vi "Synthetic_Jet_Measurement_v2.vi"() -> (5 "Plug in titles":string[](array[string]), 7 "Plug in values":string[](array[string]))   [LabVIEW 2011]
uses:
  Controls/SJ_Channels.ctl
  Controls/SJ_Data_Cluster.ctl
  <vilib>/Analysis/2dsp.llb/Integral Method.ctl
  Globals/Meas_global.vi
  Globals/Plug_in_data_global.vi
  <vilib>/Analysis/baseanly.llb/Scale 1D.vi
  <vilib>/Analysis/5stat.llb/RMS (DBL).vi
  <vilib>/Analysis/8numeric.llb/1D Numeric Integration.vi
  <vilib>/Analysis/baseanly.llb/Quick Scale 1D.vi
  <vilib>/Analysis/1siggen.llb/Ramp Pattern by Samples.vi
  <vilib>/Analysis/NI_AALBase.lvlib
  <vilib>/Analysis/NI_AALPro.lvlib
panel:
  out "Phase Average?":bool
  out "Samps per cyle":i32
  in  "Synthetic Jet Specific Channels":T1=["Synthetic_Jet:Orifice:Volume", "Synthetic_Jet:Orifice:Height", "Synthetic_Jet:Orifice:Diameter", "Synthetic_Jet:Cavity:Volume", "Synthetic_Jet:Cavity:Height", "Synthetic_Jet:Cavity:Diameter", "Synthetic_Jet:Samples:Per_Cycle", "Synthetic_Jet:Dwell:Time", "Synthetic_Jet:Minimum:Frequency", "Synthetic_Jet:Maximum:Frequency", "Synthetic_Jet:Minimum:Amplitude", "Synthetic_Jet:Maximum:Amplitude", "Synthetic_Jet:Amplitude:Delta", "Synthetic_Jet:Frequency:Delta", "Synthetic_Jet:Calibration:Velocity", "Synthetic_Jet:Calibration:Max_Amplitude", "Synthetic_Jet:Calibration:Active?", "Synthetic_Jet:Calibration:No_Of_Gens", "Synthetic_Jet:Optimisation:Switch", "Synthetic_Jet:Identification:Number"]
  out "Formation Criteria":dbl
  out "Jet Formation":bool
  out "Strouhal Number":dbl
  out "Stokes Number":dbl
  out "nu":dbl=1.55e-05
  out "Omega":dbl=1200.0
  out "Reynolds Number":dbl
  out "Charicteristic Velocity m_s":dbl
  out "Stroke Length _m_":dbl
  out "DL:Frequency":dbl=2.802671520827615
  out "Cavity:Helmholtz:Hz":dbl=428.16291209383184
  out "DL:Radius":dbl
  out "DL:Streamwise:Position":dbl=5.0
  out "LEM Velocity _ms_":dbl[](array[numeric])=[3.7049856348371377, 3.4607988115264297, 3.0653584733968287, 2.5359472607578692, 1.895702983998723, 1.1726073902466658, 0.3982632267462864, -0.3934869508418966, -1.1680398605184126, -1.8915438234131698, -2.5323782445904723, -3.062535584780142, -3.458845424238726, -3.7039871212762807, -3.787246807411894, -3.7049856348371377, -3.4607988115264297, -3.0653584733968295, -2.5359472607578692, -1.8957029839987247, -1.172607390246666, -0.3982632267462887, 0.3934869508418962, 1.1680398605184101, 1.8915438234131694, 2.53237824459047, 3.0625355847801417, 3.4588454242387248, 3.7039871212762803, 3.7872468074118935]
  out "LEM Max Velocity _ms_":dbl=3.7872475686779676
  out "LEM Phase Velocity _deg_":dbl=-258.0363282123533
  out "Phase Power _deg_":dbl=-1216.295394809798
  out "Phase Current _deg_":dbl=114.2968039724566
  out "RV Phase Pressure _deg_":dbl
  out "Phase Pressure _deg_":dbl=-169.14507601114087
  out "Phase Displ _deg_":dbl=-40.709415815185025
  out "Phase Velocity _deg_":dbl=373.1272896341652
  out "Phase Input Voltage _deg_":dbl=8.606071626556414
  out "Phase Angle _deg_":dbl[](array[numeric])=[0.0, 12.0, 24.0, 36.0, 48.0, 60.0, 72.0, 84.0, 96.0, 108.0, 120.0, 132.0, 144.0, 156.0, 168.0, 180.0, 192.0, 204.0, 216.0, 228.0, 240.0, 252.0, 264.0, 276.0, 288.0, 300.0, 312.0, 324.0, 336.0, 348.0]
  out "Max Power _W_":dbl=0.09567394666235574 format="%0.2f"
  out "Amplitude (V)":dbl=70.0
  out "Frequency (Hz)":dbl=1200.0
  out "AS Freq":dbl=36036.04
  out "Output Data Names":string[](array[string])=["Max Pressure _Pa_", "Max Velocity m_s", "Max Current _A_", "Max Displacement _m_", "Phase Displ _deg_", "Phase Pressure _deg_", "Phase Velocity _deg_", "Phase Current _deg_", "Phase Input Voltage _deg_", "LEM Max Velocity _ms_", "LEM Phase Velocity _deg_"]
  out "Current _A_":dbl[](array[numeric])=[0.007871578951352444, 0.008266417140890889, 0.00849968074403876, 0.008455354076272185, 0.007734598407207069, 0.006567672714377243, 0.00502412226480415, 0.003160545427498193, 0.0011561900642313688, -0.0008322812950871137, -0.0026496409136783387, -0.004250177970402979, -0.0056599044207173484, -0.006974613805967722, -0.007544462997563997, -0.008243629249997945, -0.008448348909812501, -0.008596065082556333, -0.008270248882544743, -0.007591372292965107, -0.0065346555924612445, -0.005182607825984795, -0.003607407527949277, -0.0016626720392260718, 0.00036386353784322137, 0.0021437834956932957, 0.003704399543557329, 0.005128068807114345, 0.006438338773620389, 0.007353635511234548]
  out "Power_W_":dbl[](array[numeric])=[-0.043363451952469156, -0.1045787042911587, -0.16349661489678932, -0.21135096948039916, -0.2294893577920496, -0.21702510361561647, -0.17587031608696657, -0.11191242161210375, -0.03966959410717387, 0.026383849953920794, 0.07342545396353153, 0.09567394666235574, 0.0925358489049179, 0.06622858320017053, 0.01657193795313242, -0.042740863570043953, -0.10421979243576313, -0.16261661392816973, -0.2041915474460092, -0.22315321729709184, -0.2143088761872366, -0.18014115682356102, -0.12703551569073906, -0.05674338994484436, 0.011476164341731257, 0.059131235834024416, 0.08299512964242624, 0.08340916969883025, 0.06053396412209597, 0.01568890358261011]
  out "RV Pressure _V_":dbl[](array[numeric])=[-14.369666524328046, -57.77058962565634, -87.07652966541758, -117.51006835010423, -142.3114261743131, -158.09199483911908, -155.83679754926837, -151.8902022920296, -142.3114261743131, -120.32906496241762, -88.20412831034297, -49.31359978871612, -12.114469234477319, 29.02544421285115, 67.35217341201532, 101.7323073539407, 128.78305010385122, 147.3826153809706, 157.5310031852989, 162.59938472331393, 149.63781267082135, 136.11244129586606, 102.29610667640338, 72.99016663664214, 42.55081558780641, -5.354689729074237, -48.18600114379076, -84.25753305310417, -116.38246970517886, -138.36483091707433, -158.65579416158175, -165.41557366698484, -160.34719212896982, -149.0712056797162, -122.58426225226835, -92.71452289004439, -56.642990980730964, -17.188663136641456, 24.515049633149694, 61.15038086492581, 97.22191277423924, 132.1658460386273, 151.3292106382094, 160.34418743346322, 160.34418743346322, 155.27580589544817, 136.67624061832876, 106.80650125610484, 74.67575223988108, 33.5358387925526, -1.9718937942981463, -42.553820283313044, -85.38513169802953, -116.38246970517886, -141.74762685185044, -159.78339280650712, -164.28797502205947, -162.03859009635784, -141.18382752938774, -123.71186089719372, -94.40592085743245, -59.46198759304437, -20.007659748954865, 21.70186538498539, 58.3313842526124, 92.14771887207513, 124.27846788829885, 149.63781267082135, 160.34418743346322, 156.9672038628362, 155.27580589544817, 141.75043452049292, 110.18348482673184, 77.49474885219449, 41.987016265343726, 0.2833034955525799, -41.42622163838768, -76.37015490277572, -109.62269019977577, -131.59923904752216, -159.21959348404445, -167.67077095683558, -160.9109914514325, -151.8902022920296, -125.96705818704444, -102.29329900776088, -63.96656980859674, -33.53303112391013, 16.627671482821253, 53.82680203706004, 93.27531751700047, 122.58706992091082, 148.51021402589598, 158.65860183022428, 155.27580589544817, 156.9672038628362, 142.30842147880648, 120.3318726310601, 80.31374546450789, 48.18880881243323, 10.425878935731753, -34.6606297688355, -76.37015490277572, -108.49509155485042, -133.85443633737287, -151.8902022920296, -162.03859009635784, -164.28797502205947, -154.709198904343, -135.54583430476092, -104.54849629761163, -71.85976032307427, -32.96923180144745, 7.0430830009556615, 52.135404069672006, 85.95173868913471, 118.64047466367205, 142.30842147880648, 157.5310031852989, 159.78038811100052, 158.09480250776156, 142.30842147880648, 123.71466856583618, 86.5155380115974, 49.316407457358586, 13.244875548045162, -27.33705094096973, -69.04076371076087, -103.42089765268625, -130.4716404025968, -151.8902022920296, -160.34719212896982, -162.60238941882054, -154.14539958188033, -135.54583430476092, -104.54849629761163, -71.85976032307427, -36.91582705868622, 4.793698075254034, 51.007805424746635, 81.44134410943326, 115.82147805135864, 140.62283587556755, 154.1482072505228, 160.9079867559259, 156.40340454037351, 145.69121741358256, 120.89567195352278, 93.27531751700047, 54.95440068198541]
  out "Displacement _m_":dbl[](array[numeric])=[-2.6563452608725367e-05, -3.3033094590941884e-05, -3.489470009695634e-05, -3.608459414033635e-05, -3.599336290251176e-05, -3.300271431749379e-05, -3.056117109155232e-05, -2.2626856342716373e-05, -1.762170629215838e-05, -1.0755312405507711e-05, -5.5370483534114006e-06, -2.8768068802271785e-07, 4.656075893275746e-06, 8.287603580077764e-06, 1.4940431377787088e-05, 1.9792866303780654e-05, 2.4126214474223672e-05, 2.519431617137013e-05, 2.644560368400959e-05, 2.7208727219429685e-05, 2.372973382223118e-05, 2.04641256790127e-05, 1.719906004067715e-05, 1.3689415117589209e-05, 8.043566800208257e-06, 4.4422385518931854e-06, -1.2338996214552368e-06, -5.841845680176716e-06, -1.1396101089811283e-05, -1.6401251140369278e-05]
  out "Input Voltage _V_":dbl[](array[numeric])=[-5.5088632433799996, -12.651031578584, -19.235618350895997, -24.9961110527, -29.670494279084004, -33.04444558276, -35.005182361704, -35.409211536216006, -34.310616683552006, -31.700640287920002, -27.711473499856005, -22.510574222680006, -16.349366000988, -9.495663135284, -2.196569584672, 5.184714435096, 12.336113665324001, 18.917564300223997, 24.689891482827996, 29.395636083331993, 32.795741589576, 34.758786092276, 35.215182844328, 34.127830748423996, 31.539748142271996, 27.582652797175996, 22.404475723135995, 16.265220463328, 9.402109185388, 2.133489422836]
  out "Pressure _Pa_":dbl[](array[numeric])=[-27.3956675953706, 95.65286233449294, 217.28142105099454, 325.3916285730047, 412.49320713856633, 477.62511872885386, 518.8812420389512, 544.5955786383588, 546.2858417945154, 525.7943338813993, 485.98446016799124, 431.53940396868336, 357.29264741860004, 257.81676584697294, 146.44897730607346, 25.39291194062997, -95.29994862668336, -216.63005998968256, -325.4638615668826, -412.65459893301875, -477.423305725176, -519.6780076017092, -543.7330519967387, -544.6659346048561, -524.568602441649, -487.2326508157636, -435.0203186855821, -361.9795522274816, -267.2741357434412, -152.01151538796677]
  out "Zeros":dbl[](array[numeric])=[1.4978743085562871, 0.2341330189017041, -0.35175473981443495, 0.0022887999999999997, -3.0068544366899315, 2.8293]
  out "Velocity m_s":dbl[](array[numeric])=[-0.006589971422005106, -0.006419643065741468, -0.009111611844261746, -0.006030326884042168, -0.004272653157727323, -0.0068849933436421745, -0.010636233235274354, -0.0035467148583991693, -0.008496862890472292, -0.005357351691532665, -0.007065956289182962, -0.006648911559621155, -0.005058171342073957, -0.008830133605031026, -0.0038751674420970687, -0.005274584307176274, 0.000979796600094568, -0.005616008146962059, -0.00729733372181674, 0.0005036149760482819, -0.004633370846616606, -0.007598533001820504, -0.005354959759266961, -0.003855515705978843, -0.005082756078867318, -0.0008163141834672163, -0.007346968606858383, -0.00413574997102441, -0.00277648312445221, -0.00052352239052674]
  out "Max Current _A_":dbl=0.00849968074403876 format="%e"
  out "RMS Dispacement _m_":dbl=2.25005755896471e-05 format="%0.2f"
  out "RMS Velocity m_s":dbl=0.014914535983039488 format="%0.2f"
  out "RMS Current _A_":dbl=0.006206722435388947 format="%0.2f"
  out "RV RMS Pressure _V_":dbl format="%0.2f"
  out "RMS Pressure _Pa_":dbl=395.7699897259115 format="%0.2f"
  out "RMS Power _W_":dbl=0.13002833315099252 format="%0.2f"
  out "Max Displacement _m_":dbl=2.7208727219429685e-05 format="%e"
  out "Max Pressure _Pa_":dbl=546.2858417945154 format="%0.2f"
  out "RV Max Pressure _V_":dbl format="%0.2f"
  out "Max Velocity m_s":dbl=0.000979796600094568
  out "Current Plot":cluster{dbl[], dbl[]}[](graph)=[{[0.0, 12.0, 24.0, 36.0, 48.0, 60.0, 72.0, 84.0, 96.0, 108.0, 120.0, 132.0, 144.0, 156.0, 168.0, 180.0, 192.0, 204.0, 216.0, 228.0, 240.0, 252.0, 264.0, 276.0, 288.0, 300.0, 312.0, 324.0, 336.0, 348.0], [-0.15557712257291065, -0.35728080433659803, -0.5432376920119246, -0.705921142218441, -0.8379315153272326, -0.9332160799164545, -0.9885897155857659, -1.0, -0.9689743203815658, -0.8952653536353687, -0.7826063416157439, -0.6357265029653804, -0.4617263500562873, -0.2681692905127802, -0.06203384626131485, 0.1464227586596542, 0.34838713233438734, 0.5342554516040381, 0.697273122209331, 0.8301691793748806, 0.926192371045399, 0.9816311796924717, 0.9945203893712923, 0.9638122191316959, 0.8907215601232357, 0.7789682853842954, 0.632730149899583, 0.45934997583022086, 0.26552721106968635, 0.060252384345070756]}, {[0.0, 12.0, 24.0, 36.0, 48.0, 60.0, 72.0, 84.0, 96.0, 108.0, 120.0, 132.0, 144.0, 156.0, 168.0, 180.0, 192.0, 204.0, 216.0, 228.0, 240.0, 252.0, 264.0, 276.0, 288.0, 300.0, 312.0, 324.0, 336.0, 348.0], [0.915718863893427, 0.9616512975995976, 0.9887873884629885, 0.9836307653638304, 0.8997836024883751, 0.7640324556993839, 0.5844676856855597, 0.36767351074525567, 0.13450224644966696, -0.09682119517406056, -0.3082388148799797, -0.49443296782707047, -0.6584296845544803, -0.8113728478069623, -0.8776647134598465, -0.9590003298982027, -0.9828158382556238, -1.0, -0.962097052909388, -0.8831217795651628, -0.7601914980520298, -0.6029046751288172, -0.41965800552972216, -0.19342245821289428, 0.04232908131205239, 0.24939125926856856, 0.4309413095387709, 0.5965600257634787, 0.7489867412341333, 0.855465313560387]}]
  in  "Menu Ring":u16(ring) items=["Max Pressure _Pa_", "Max Velocity m_s", "Max Current _A_", "Max Displacement _m_", "Phase Displ _deg_", "Phase Pressure _deg_", "Phase Velocity _deg_", "Phase Current _deg_", "Phase Input Voltage _deg_", "LEM Max Velocity _ms_", "LEM Phase Velocity _deg_"]
  out "Pressure v Frequency":cluster{dbl[], dbl[]}(graph)
  out "Pressure Plot":cluster{dbl[], dbl[]}[](graph)=[{[0.0, 12.0, 24.0, 36.0, 48.0, 60.0, 72.0, 84.0, 96.0, 108.0, 120.0, 132.0, 144.0, 156.0, 168.0, 180.0, 192.0, 204.0, 216.0, 228.0, 240.0, 252.0, 264.0, 276.0, 288.0, 300.0, 312.0, 324.0, 336.0, 348.0], [-0.15557712257291065, -0.35728080433659803, -0.5432376920119246, -0.705921142218441, -0.8379315153272326, -0.9332160799164545, -0.9885897155857659, -1.0, -0.9689743203815658, -0.8952653536353687, -0.7826063416157439, -0.6357265029653804, -0.4617263500562873, -0.2681692905127802, -0.06203384626131485, 0.1464227586596542, 0.34838713233438734, 0.5342554516040381, 0.697273122209331, 0.8301691793748806, 0.926192371045399, 0.9816311796924717, 0.9945203893712923, 0.9638122191316959, 0.8907215601232357, 0.7789682853842954, 0.632730149899583, 0.45934997583022086, 0.26552721106968635, 0.060252384345070756]}, {[0.0, 12.0, 24.0, 36.0, 48.0, 60.0, 72.0, 84.0, 96.0, 108.0, 120.0, 132.0, 144.0, 156.0, 168.0, 180.0, 192.0, 204.0, 216.0, 228.0, 240.0, 252.0, 264.0, 276.0, 288.0, 300.0, 312.0, 324.0, 336.0, 348.0], [-0.05014896140338823, 0.1750967259562854, 0.39774309423293575, 0.5956435325215701, 0.7550867615085017, 0.8743135592895557, 0.9498346878887768, 0.9969058997564276, 1.0, 0.9624894032658751, 0.8896156974736197, 0.7899516534258018, 0.6540397353973438, 0.47194480640402603, 0.2680812243366908, 0.0464828300459258, -0.17445070206035157, -0.39655074947222896, -0.5957757581594167, -0.7553821962097238, -0.87394413180629, -0.9512932019153176, -0.9953270072140422, -0.9970346894139926, -0.9602456485390019, -0.8919005647578826, -0.7963236192550169, -0.6626193185574809, -0.4892569334498257, -0.2782636922981901]}]
  out "Displacement Plot":cluster{dbl[], dbl[]}[](graph)=[{[0.0, 12.0, 24.0, 36.0, 48.0, 60.0, 72.0, 84.0, 96.0, 108.0, 120.0, 132.0, 144.0, 156.0, 168.0, 180.0, 192.0, 204.0, 216.0, 228.0, 240.0, 252.0, 264.0, 276.0, 288.0, 300.0, 312.0, 324.0, 336.0, 348.0], [-0.15557712257291065, -0.35728080433659803, -0.5432376920119246, -0.705921142218441, -0.8379315153272326, -0.9332160799164545, -0.9885897155857659, -1.0, -0.9689743203815658, -0.8952653536353687, -0.7826063416157439, -0.6357265029653804, -0.4617263500562873, -0.2681692905127802, -0.06203384626131485, 0.1464227586596542, 0.34838713233438734, 0.5342554516040381, 0.697273122209331, 0.8301691793748806, 0.926192371045399, 0.9816311796924717, 0.9945203893712923, 0.9638122191316959, 0.8907215601232357, 0.7789682853842954, 0.632730149899583, 0.45934997583022086, 0.26552721106968635, 0.060252384345070756]}, {[0.0, 12.0, 24.0, 36.0, 48.0, 60.0, 72.0, 84.0, 96.0, 108.0, 120.0, 132.0, 144.0, 156.0, 168.0, 180.0, 192.0, 204.0, 216.0, 228.0, 240.0, 252.0, 264.0, 276.0, 288.0, 300.0, 312.0, 324.0, 336.0, 348.0], [-0.7361438653132033, -0.9154348379941063, -0.9670248738630008, -1.0, -0.997471739948916, -0.9145929198799676, -0.8469312685822951, -0.6270503211070746, -0.48834431180314575, -0.2980582894650082, -0.15344632481876624, -0.00797239638899362, 0.12903223672595104, 0.2296715198692966, 0.4140390583217413, 0.5485129256769343, 0.668601519540294, 0.6982014560947281, 0.7328779584207091, 0.7540261396210363, 0.6576139870090829, 0.5671153068654675, 0.47663166097388826, 0.3793700731217815, 0.22290861216080401, 0.12310623571424707, -0.03419463765219268, -0.16189306875552578, -0.3158162468307329, -0.45452225613466185]}]
  out "Velocity Plot":cluster{dbl[], dbl[]}[](graph)=[{[0.0, 12.0, 24.0, 36.0, 48.0, 60.0, 72.0, 84.0, 96.0, 108.0, 120.0, 132.0, 144.0, 156.0, 168.0, 180.0, 192.0, 204.0, 216.0, 228.0, 240.0, 252.0, 264.0, 276.0, 288.0, 300.0, 312.0, 324.0, 336.0, 348.0], [-0.15557712257291065, -0.35728080433659803, -0.5432376920119246, -0.705921142218441, -0.8379315153272326, -0.9332160799164545, -0.9885897155857659, -1.0, -0.9689743203815658, -0.8952653536353687, -0.7826063416157439, -0.6357265029653804, -0.4617263500562873, -0.2681692905127802, -0.06203384626131485, 0.1464227586596542, 0.34838713233438734, 0.5342554516040381, 0.697273122209331, 0.8301691793748806, 0.926192371045399, 0.9816311796924717, 0.9945203893712923, 0.9638122191316959, 0.8907215601232357, 0.7789682853842954, 0.632730149899583, 0.45934997583022086, 0.26552721106968635, 0.060252384345070756]}, {[0.0, 12.0, 24.0, 36.0, 48.0, 60.0, 72.0, 84.0, 96.0, 108.0, 120.0, 132.0, 144.0, 156.0, 168.0, 180.0, 192.0, 204.0, 216.0, 228.0, 240.0, 252.0, 264.0, 276.0, 288.0, 300.0, 312.0, 324.0, 336.0, 348.0], [-0.0017400427690923374, -0.0016950685794170583, -0.002405866928563968, -0.0015922719565676093, -0.001128168660507009, -0.0018179415532591603, -0.002808434141249664, -0.0009364889690996669, -0.002243546122698781, -0.0014145768585897204, -0.0018657237429983216, -0.001755605561963586, -0.0013355800662831847, -0.0023315442732039188, -0.0010232149208002786, -0.001392722622896813, 0.00025870946624789303, -0.0014828735576385352, -0.0019268175782828233, 0.00013297653986074366, -0.0012234140213805954, -0.002006347457194939, -0.0014139452830977239, -0.0010180259967302217, -0.001342071519849202, -0.00021554290622666447, -0.0019399233745421283, -0.001092020188103525, -0.0007331138596561618, -0.00013823297428152076]}, {[0.0, 12.0, 24.0, 36.0, 48.0, 60.0, 72.0, 84.0, 96.0, 108.0, 120.0, 132.0, 144.0, 156.0, 168.0, 180.0, 192.0, 204.0, 216.0, 228.0, 240.0, 252.0, 264.0, 276.0, 288.0, 300.0, 312.0, 324.0, 336.0, 348.0], [0.9782794265180274, 0.9138033477917035, 0.8093896778519208, 0.6696017951074252, 0.5005491008108334, 0.3096200089077361, 0.10515903689372944, -0.10389788964157722, -0.3084139798421589, -0.49945089918916635, -0.6686594176102914, -0.8086443108979737, -0.9132875674934984, -0.9780157749495838, -1.0, -0.9782794265180274, -0.9138033477917035, -0.8093896778519211, -0.6696017951074252, -0.5005491008108338, -0.30962000890773617, -0.10515903689373006, 0.10389788964157712, 0.3084139798421583, 0.4994508991891662, 0.6686594176102908, 0.8086443108979736, 0.9132875674934979, 0.9780157749495837, 0.9999999999999999]}]
  out "Amplitude String":string="3.5000"
  out "Frequency String":string="1200"
  # "You Must have selected the \"Save Data\" option on the \nMeasurement Program for this vi to work correctly"
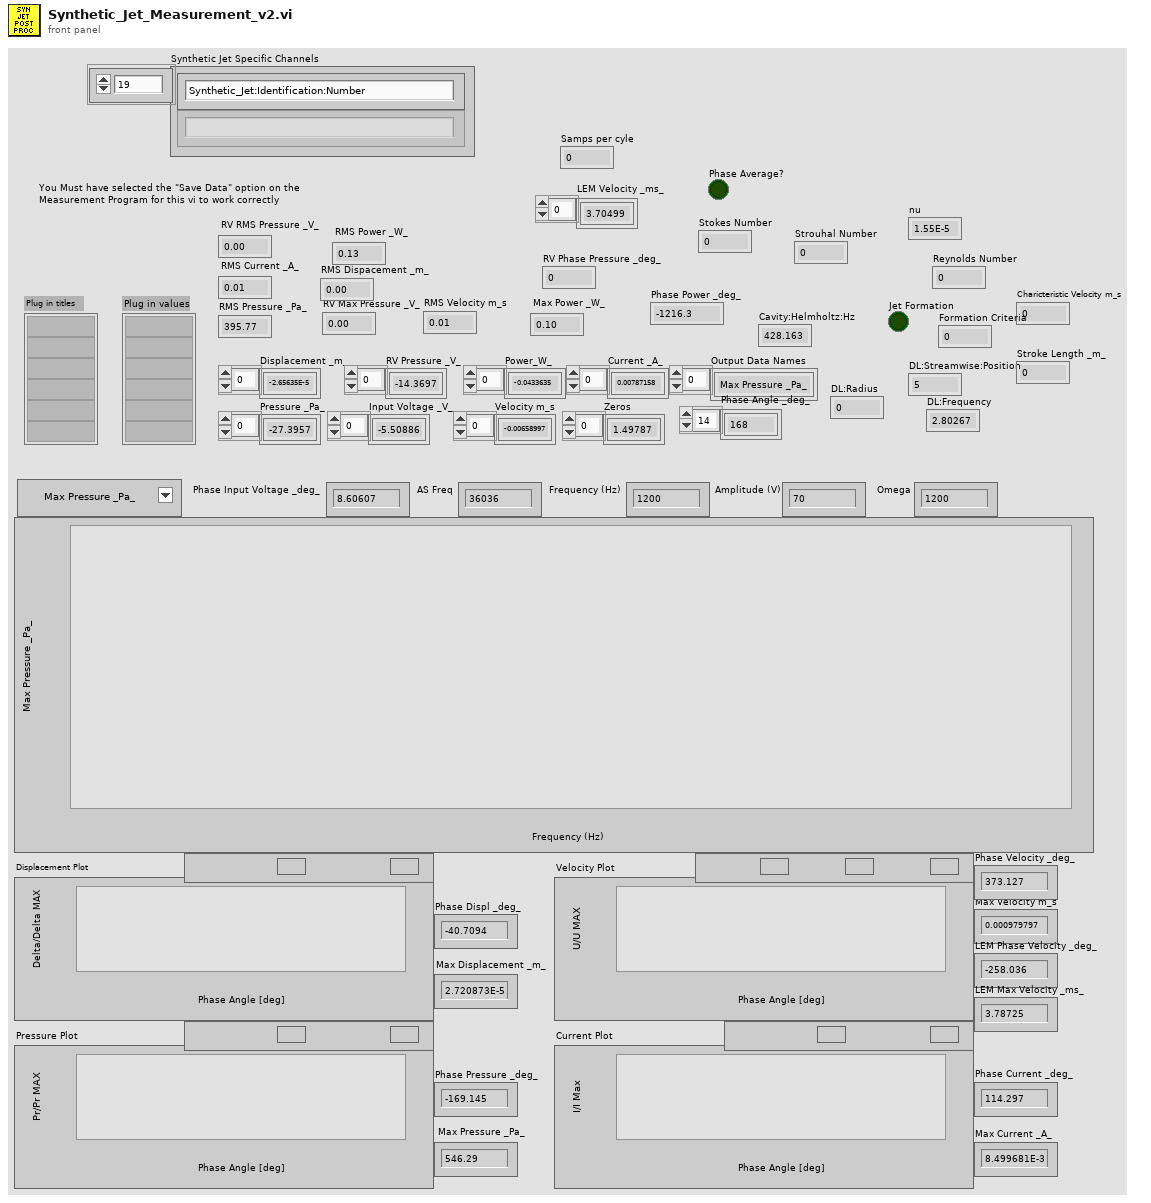
[diagram p1: front panel]
types:
  T1 = typedef "SJ_Channels.ctl" = string[]
  T2 = typedef "Analysis_info_cluster.ctl" = cluster{"Colour":u32, "Inst type":T3, "Inst name":string, "Symbol":string, "Code name":string, "Extra Info":string, "Inst Array":T4, "Index":i32, "Voltage Index":i32, "Extra Titles":string[], "Extra Values":string[]}
  T3 = typedef "Inst_type.ctl" = enum16{"Propeller anemometer", "Raw voltage", "Pressure Transducer", "Pitot-static tube", "Preston tube", "Hot wire", "Cross wire 1", "Cross wire 2", "Generic Linear", "Generic Polynomial", "Generic BackPoly", "Fast FID", "Thermocouple", "Cold wire", "Pulsed Wire", "LDA Vel", "LDA Tran time", "LDA Arr time"}
  T4 = typedef "Instrument_Array.ctl" = enum16{"PWA", "LDA", "Analogue"}
  T5 = typedef "Post_Process.ctl" = enum16{"Take New Data", "Post Process Raw Data File"}
  T6 = cluster{"Name":string, "X":dbl, "Y":dbl, "Z":dbl}[]
  T7 = typedef "SJ_Data_Cluster.ctl" = cluster{"Do":dbl, "Dc":dbl, "Ho":dbl, "Hc":dbl, "K":dbl, "beta":dbl, "Vc":dbl, "Vo":dbl}
  T8 = cluster{"R":dbl, "Mair":dbl, "T":dbl, "Patmos":dbl, "gamma":dbl}
  T9 = cluster{"Name":string, "X":dbl, "Y":dbl, "Z":dbl}
  T10 = typedef "NI_AALPro.lvlib/Integral Method.ctl" = i32
  T11 = cluster{"Ramp Pattern":dbl[], "Y[i]=X[i]/Max|X|":dbl[]}
  T12 = cluster{"Ramp Pattern":dbl[], "Y[i]=X[i]/Max|X|":dbl[]}[]
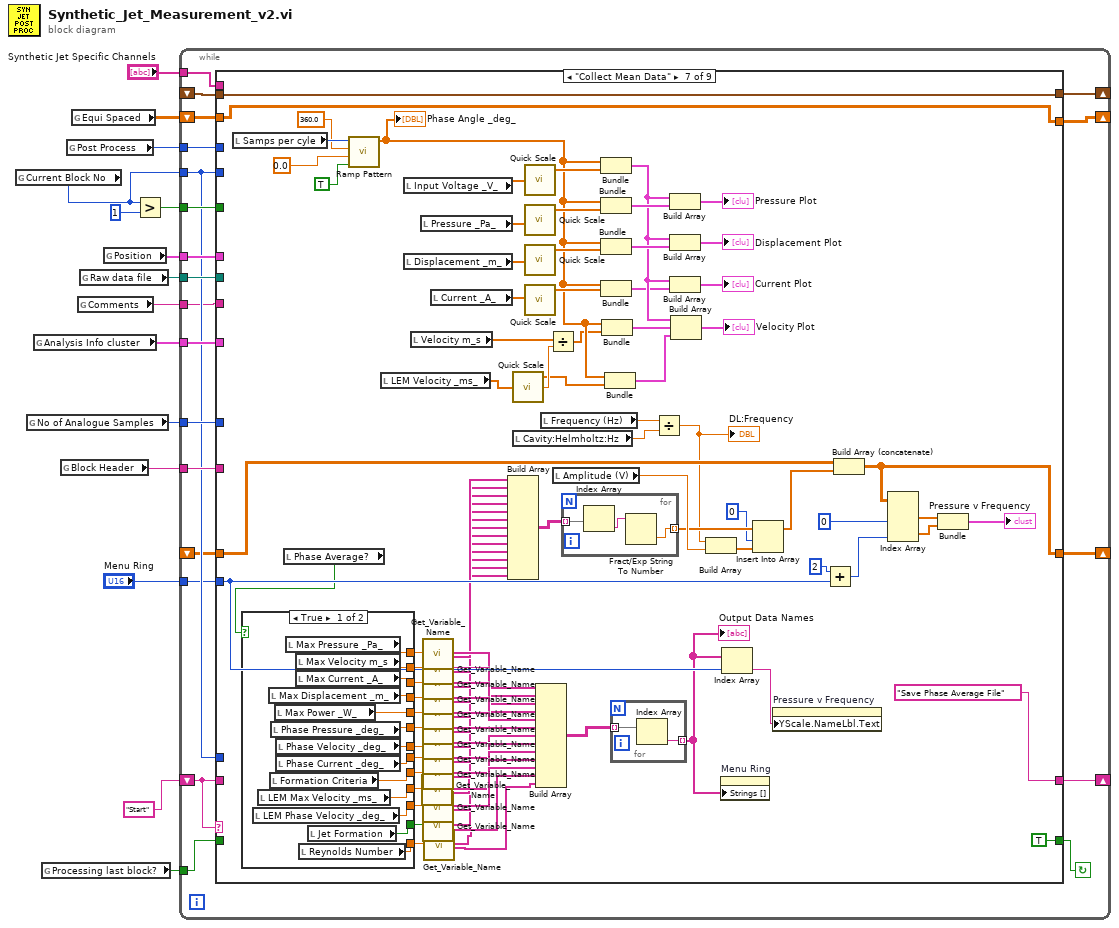
[diagram p0: block diagram]
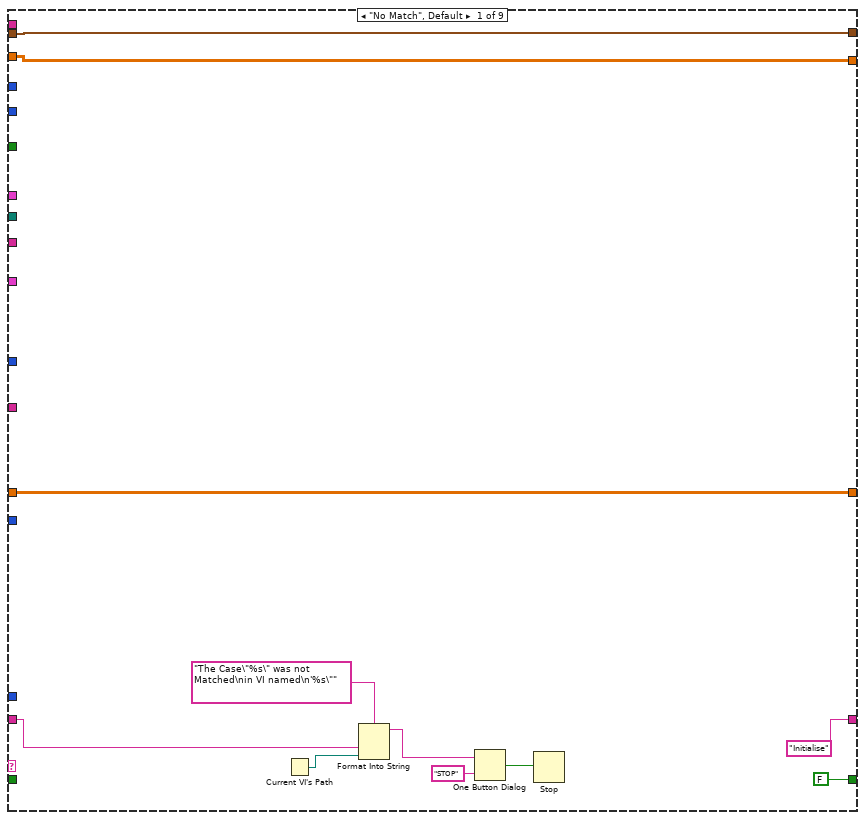
[diagram p2: hidden frame]
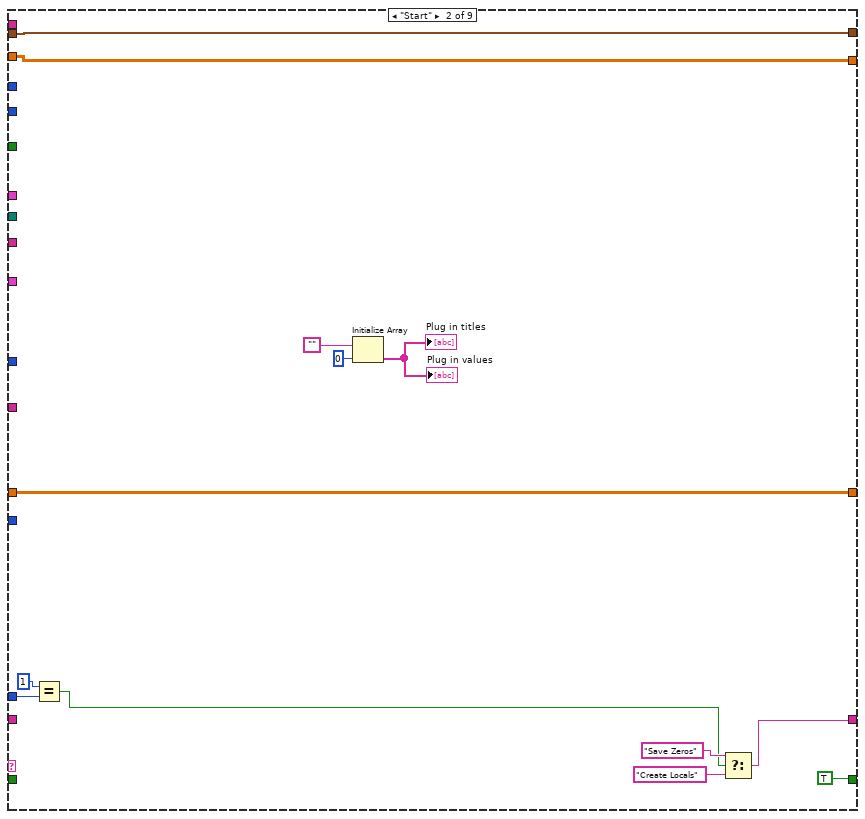
[diagram p3: hidden frame]
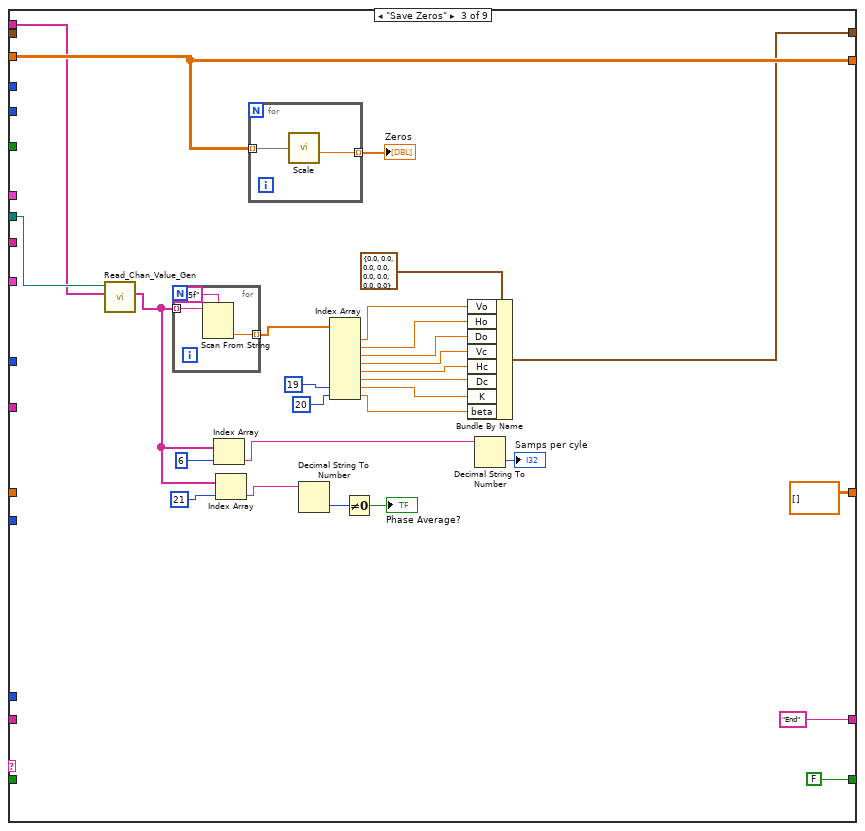
[diagram p4: hidden frame]
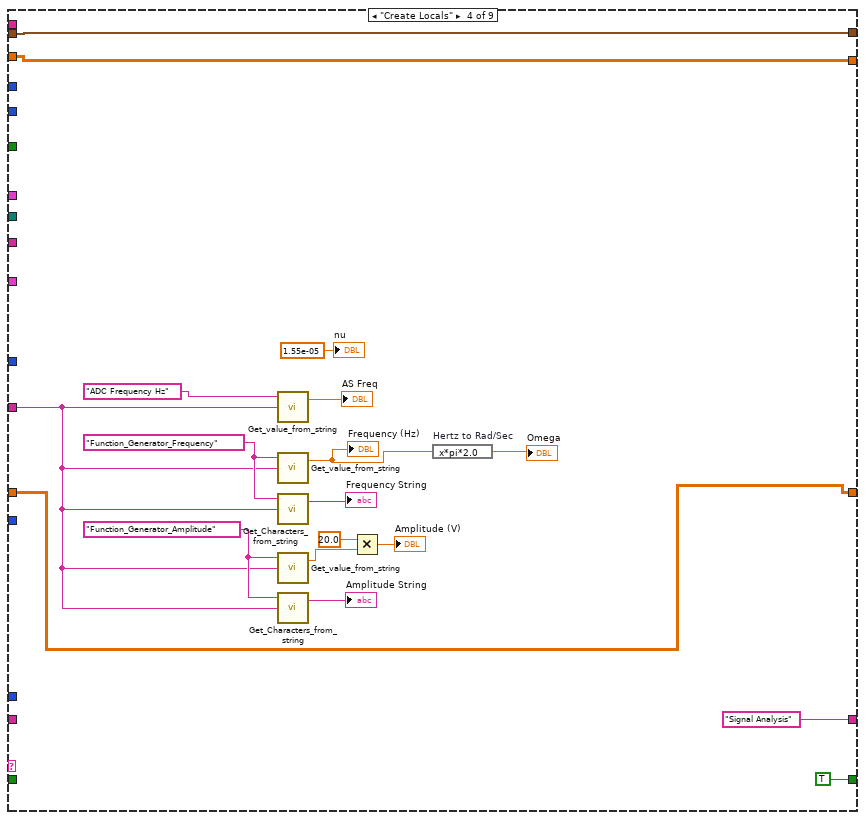
[diagram p5: hidden frame]
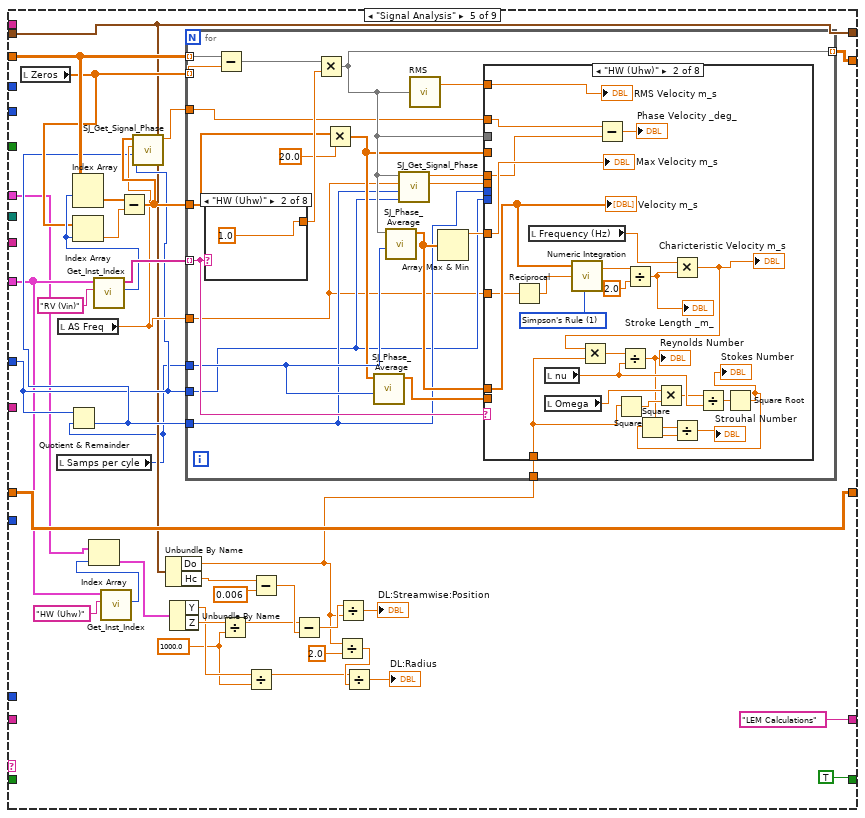
[diagram p6: hidden frame]
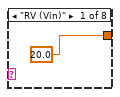
[diagram p7: hidden frame]
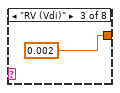
[diagram p8: hidden frame]
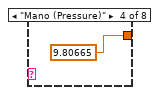
[diagram p9: hidden frame]
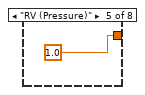
[diagram p10: hidden frame]
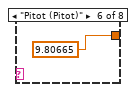
[diagram p11: hidden frame]
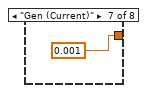
[diagram p12: hidden frame]
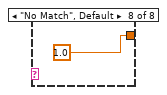
[diagram p13: hidden frame]
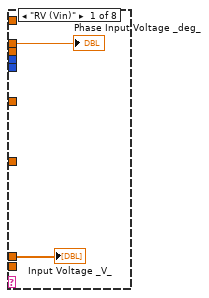
[diagram p14: hidden frame]
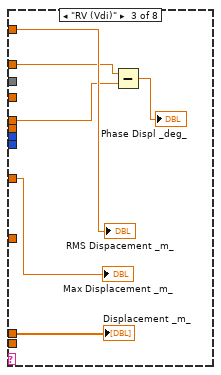
[diagram p15: hidden frame]
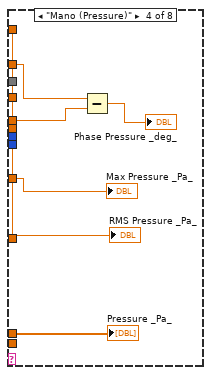
[diagram p16: hidden frame]
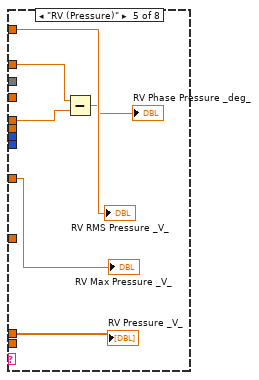
[diagram p17: hidden frame]
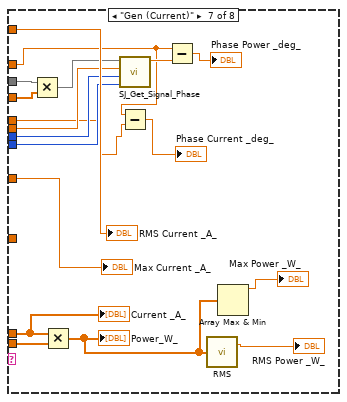
[diagram p19: hidden frame]
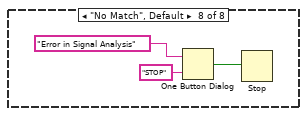
[diagram p20: hidden frame]
diagram:
  n1 = global read "Meas_global.vi" "Current Block No"() -> (w11:i32)
  n2 = global read "Meas_global.vi" "No of Analogue Samples"() -> (w7:i32)
  n3 = global read "Meas_global.vi" "Analysis Info cluster"() -> (w10:T2[])
  n4 = global read "Meas_global.vi" "Processing last block?"() -> (w5:bool)
  n5 = global read "Plug_in_data_global.vi" "Block Header"() -> (w8:string)
  n6 = global read "Meas_global.vi" "Post Process"() -> (w2:T5)
  n7 = global read "Plug_in_data_global.vi" "Equi Spaced"() -> (w9:dbl[][])
  n8 = global read "Meas_global.vi" "Comments"() -> (w4:string)
  n9 = global read "Meas_global.vi" "Raw data file"() -> (w14:path)
  n10 = global read "Meas_global.vi" "Position"() -> (w6:T6)
  n11 = Greater?(x=w11, y=1) -> (0:w12:bool)
  n12 = while {
    shift-left: "Start" -> [w36]
    shift-right: [w26] -> _
    tunnel: w14 -> [w35]
    tunnel: w12 -> [w34]
    tunnel: w11 -> [w27]
    tunnel: w10 -> [w33]
    tunnel: w8 -> [w31]
    tunnel: w7 -> [w30]
    tunnel: w6 -> [w29]
    tunnel: w5 -> [w28]
    shift-right: [w24] -> _
    shift-left: w9 -> [w32]
    shift-right: [w23] -> _
    shift-left: _ -> [w22]
    tunnel: w4 -> [w21]
    tunnel: "Menu Ring" -> [w20]
    tunnel: w2 -> [w19]
    shift-right: [w17] -> _
    shift-left: _ -> [w18]
    tunnel: "Synthetic Jet Specific Channels" -> [w16]
    stop <- w25 continue-if-true
    n13 = case shown="\"Collect Mean Data\"" w36 {
      tunnel: w36 -> [w43 _ _ _ _ _ _ _ _]
      tunnel: w35 -> [_ _ w81 _ _ w249 _ w474 w525]
      tunnel: w34 -> [_ _ _ _ _ _ _ _ _]
      tunnel: w27 -> [_ _ _ _ _ _ _ _ _]
      tunnel: w33 -> [_ _ _ _ w131 _ _ _ _]
      tunnel: w32 -> [w39 w51 w85 w103 w139 w269 w327 w472 w578]
      tunnel: w31 -> [_ _ _ w106 _ _ _ _ _]
      tunnel: w30 -> [_ _ _ _ w134 _ _ _ _]
      tunnel: w29 -> [_ _ _ _ w130 _ _ _ _]
      tunnel: w28 -> [_ _ _ _ _ _ _ w400 _]
      tunnel: w27 -> [_ w57 _ _ _ _ _ _ _]
      tunnel: ["Initialise" w53 "End" ("t") "Signal Analysis" "LEM Calculations" "Collect Mean Data" "Save Phase Average File" "Save Mean Data" ("t") "End"] -> w26
      tunnel: [FALSE TRUE FALSE TRUE TRUE TRUE ("Processing last block?") TRUE ("Processing last block?") w400 FALSE ("Processing last block?")] -> w25
      tunnel: [w39 w51 w85 w103 w146 w269 w327 w472 w578] -> w24
      tunnel: [w38 w50 dbl[][] [] w102 w143 w273 w358 w413 w570] -> w23
      tunnel: w22 -> [w38 w50 _ w102 w143 w273 w359 w413 w570]
      tunnel: w21 -> [_ _ _ _ _ _ _ w415 w544]
      tunnel: w20 -> [_ _ _ _ _ _ w333 _ _]
      tunnel: w19 -> [_ _ _ _ _ _ _ _ _]
      tunnel: w18 -> [w37 w48 _ w94 w127 w253 w291 w427 w569]
      tunnel: [w37 w48 w82 w94 w127 w253 w291 w427 w569] -> w17
      tunnel: w16 -> [_ _ w80 _ _ _ _ _ _]
      frame "No Match", Default {
        n14 = Current VI's Path() -> (path=w42:path)
        n15 = Format Into String(format string="The Case\"%s\" was not Matched\nin VI named\n'%s\"" ("Format String"), w43, w42) -> (resulting string=w46:string)  [unwired: 2 in, 1 out]
        n16 = One Button Dialog(message=w46, button name ("OK")="STOP") -> (true=w44:bool)
        n17 = Stop(stop? (T)=w44) -> ()
      }
      frame "Start" {
        n18 = Equal?(x=1, y=w57) -> (x = y?=w49:bool)
        n19 = Initialize Array("", 0) -> (→"Plug in values" →"Plug in titles":string[])
        n20 = Select(t="Save Zeros", s=w49, f="Create Locals") -> (s? t:f=w53:string)
      }
      frame "Save Zeros" {
        (unwired) FALSE ("Processing last block?")
        (unwired) "End" ("t")
        (unwired) "End" ("t")
        (unwired) FALSE ("Processing last block?")
        n21 = call "Read_Chan_Value_Gen.vi"("Desired Ch Names"=w80, "Raw data file"=w81) -> ("Values"=w64:string[])  [unwired: 9 in]
        n22 = for {
          tunnel: w64 -> [w91] mode=indexing
          tunnel: [w89] -> w69 mode=indexing
          n23 = Scan From String(format string="%5f", input string=w91) -> (output 1=w89:dbl)  [unwired: 3 in, 3 out]
        }
        n24 = Index Array(array=w64, index=6) -> (element=w67:string)
        n25 = Index Array(array=w64, index=21) -> (element=w63:string)
        n26 = for {
          tunnel: w85 -> [w93] mode=indexing
          tunnel: [w92] -> w87 mode=indexing
          n27 = call-poly <vilib>:"Scale.vi"("X"=w93) -> ("offset"=w92:dbl)  [unwired: 3 out]
        }
        "Zeros" <- w87
        n28 = Decimal String To Number(string=w63) -> (number=w62:i32)  [unwired: 2 in, 1 out]
        n29 = Index Array(array=w69, index #7=19 ("index"), index #8=20 ("index")) -> (element #1=w79:dbl, element #2=w78:dbl, element #3=w77:dbl, element #4=w76:dbl, element #5=w75:dbl, element #6=w74:dbl, element #7=w71:dbl, element #8=w70:dbl)  [unwired: 6 in]
        n30 = Not Equal To 0?(x=w62) -> (x != 0?=→"Phase Average?":bool)
        n31 = Bundle By Name(cluster=T7 {"Do"=0.0, "Dc"=0.0, "Ho"=0.0, "Hc"=0.0, "K"=0.0, "beta"=0.0, "Vc"=0.0, "Vo"=0.0} ("SJ_Data_Cluster"), "Vo"=w79, "Ho"=w78, "Do"=w77, "Vc"=w76, "Hc"=w75, "Dc"=w74, "K"=w71, "beta"=w70) -> (w82:T7)
        n32 = Decimal String To Number(string=w67) -> (number=→"Samps per cyle":i32)  [unwired: 2 in, 1 out]
      }
      frame "Create Locals" {
        w108 = "Function_Generator_Amplitude" ("Variable name")
        w109 = "Function_Generator_Frequency" ("Variable name")
        n33 = call "Get_value_from_string.vi"("Input string"=w106, "Variable name"="ADC Frequency Hz") -> ("Value"=→"AS Freq":dbl)  [unwired: 1 in, 1 out]
        n34 = call "Get_value_from_string.vi"("Input string"=w106, "Variable name"=w109) -> ("Value"=w97:dbl)  [unwired: 1 in, 1 out]
        "Frequency (Hz)" <- w97
        n35 = call "Get_Characters_from_string.vi"("Input string"=w106, "Variable name"=w109) -> ("Value"=→"Frequency String":string)  [unwired: 1 in, 1 out]
        n36 = call "Get_value_from_string.vi"("Input string"=w106, "Variable name"=w108) -> ("Value"=w100:dbl)  [unwired: 1 in, 1 out]
        n37 = call "Get_Characters_from_string.vi"("Input string"=w106, "Variable name"=w108) -> ("Value"=→"Amplitude String":string)  [unwired: 1 in, 1 out]
        n38 = Multiply(x=20.0, y=w100) -> (x*y=→"Amplitude (V)":dbl)
        n39 = expression code="x*pi*2.0" "Hertz to Rad/Sec"(w97) -> (→"Omega":dbl)
        "nu" <- 1.55e-05 ("y")
      }
      frame "Signal Analysis" {
        w114 = 1000.0 ("y")
        n40 = local read "Zeros"() -> (w138:dbl[])
        n41 = local read "Samps per cyle"() -> (w112:i32)
        n42 = local read "AS Freq"() -> (w136:dbl)
        n43 = Quotient & Remainder(x=w134, y=w112) -> (floor(x/y)=w135:i32)  [unwired: 1 out]
        n44 = call "Get_Inst_Index.vi"("Inst name search"="RV (Vin)" ("element"), "Analysis Info cluster"=w131) -> ("Index of Instance"=w140:i32, "Inst Name Array"=w144:string[])  [unwired: 7 in, 1 out]
        n45 = Index Array(array=w139, index (row)=w140) -> (element=w141:dbl[])  [unwired: 1 in]
        n46 = Index Array(array=w138, index=w140) -> (element=w142:dbl)
        n47 = call "Get_Inst_Index.vi"("Inst name search"="HW (Uhw)" ("element"), "Analysis Info cluster"=w131) -> ("Index of Instance"=w129:i32)  [unwired: 7 in, 2 out]
        n48 = Index Array(array=w130, index=w129) -> (element=w128:T9)
        n49 = Subtract(x=w141, y=w142) -> (x-y=w137:dbl[])
        n50 = call "SJ_Get_Signal_Phase.vi"("No of Analogue Samples"=w134, "Number of Cycles"=w135, "Actual Sampling Frequency"=w136, "Signal"=w137) -> ("Phase Angle _deg_"=w133:dbl)  [unwired: 7 in]
        n51 = Unbundle By Name(w127) -> ("Do"=w113:dbl, "Hc"=w126:dbl)
        n52 = Unbundle By Name(w128) -> ("Y"=w118:dbl, "Z"=w123:dbl)
        n53 = for {
          tunnel: w139 -> [w168] mode=indexing
          tunnel: w138 -> [w167] mode=indexing
          tunnel: [w156] -> w146 mode=indexing
          tunnel: w144 -> [w165] mode=indexing
          tunnel: w112 -> [w158]
          tunnel: w136 -> [w150]
          tunnel: w134 -> [w153]
          tunnel: w135 -> [w154]
          tunnel: w137 -> [w152]
          tunnel: w133 -> [w151]
          tunnel: w113 -> [w149]
          n54 = case shown="\"HW (Uhw)\"" w165 {
            tunnel: [20.0 1.0 0.002 9.80665 1.0 9.80665 0.001 1.0] -> w163
            frame "RV (Vin)" {
            }
            frame "HW (Uhw)" {
            }
            frame "RV (Vdi)" {
            }
            frame "Mano (Pressure)" {
            }
            frame "RV (Pressure)" {
            }
            frame "Pitot (Pitot)" {
            }
            frame "Gen (Current)" {
            }
            frame "No Match", Default {
            }
          }
          n55 = Subtract(x=w168, y=w167) -> (x-y=w166:dbl[])
          n56 = Multiply(x=w166, y=w163) -> (x*y=w156:dbl[])
          n57 = Multiply(x=w152, y=20.0) -> (x*y=w155:dbl[])
          n58 = call "SJ_Phase_Average.vi"("No. of Bins"=w158, "1D Signal"=w155) -> ("Phase Averaged Signal"=w161:dbl[])  [unwired: 7 in, 2 out]
          n59 = call "SJ_Phase_Average.vi"("No. of Bins"=w158, "1D Signal"=w156) -> ("Phase Averaged Signal"=w160:dbl[])  [unwired: 7 in, 2 out]
          n60 = call "SJ_Get_Signal_Phase.vi"("No of Analogue Samples"=w153, "Number of Cycles"=w154, "Actual Sampling Frequency"=w150, "Signal"=w156) -> ("Phase Angle _deg_"=w157:dbl)  [unwired: 7 in]
          n61 = call-poly <vilib>:"RMS.vi"("X"=w156) -> ("rms value"=w164:dbl)  [unwired: 1 out]
          n62 = Array Max & Min(array=w160) -> (max value=w159:dbl)  [unwired: 3 out]
          n63 = case shown="\"HW (Uhw)\"" w165 {
            tunnel: w160 -> [w178 w198 w209 w215 w221 _ w238 _]
            tunnel: w161 -> [_ _ _ _ _ _ w239 _]
            tunnel: w164 -> [_ w203 w208 w214 w220 _ w236 _]
            tunnel: w159 -> [_ w202 w207 w213 w219 _ w235 _]
            tunnel: w157 -> [w177 w201 w205 w211 w217 _ w224 _]
            tunnel: w156 -> [_ _ _ _ _ _ w232 _]
            tunnel: w155 -> [_ _ _ _ _ _ w231 _]
            tunnel: w150 -> [_ _ _ _ _ _ w229 _]
            tunnel: w154 -> [_ _ _ _ _ _ w228 _]
            tunnel: w153 -> [_ _ _ _ _ _ w227 _]
            tunnel: w151 -> [_ w200 w204 w212 w218 _ w222 _]
            tunnel: w150 -> [_ w196 _ _ _ _ _ _]
            tunnel: w149 -> [_ w187 _ _ _ _ _ _]
            frame "RV (Vin)" {
              "Input Voltage _V_" <- w178
              "Phase Input Voltage _deg_" <- w177
            }
            frame "HW (Uhw)" {
              w197 = T10 1 items=["Trapezoidal Rule", "Simpson's Rule", "Simpson's 3/8 Rule", "Bode Rule"] ("integration method")
              n64 = Reciprocal(x=w196) -> (1/x=w195:dbl)
              n65 = local read "Frequency (Hz)"() -> (w191:dbl)
              n66 = local read "nu"() -> (w185:dbl)
              n67 = local read "Omega"() -> (w186:dbl)
              n68 = call-poly <vilib>:"Numeric Integration.vi"("integration method"=w197, "dt"=w195, "Input Array"=w198) -> ("result"=w194:dbl)  [unwired: 1 out]
              n69 = Subtract(x=w200, y=w201) -> (x-y=→"Phase Velocity _deg_":dbl)
              n70 = Square(x=w187) -> (x^2=w188:dbl)
              n71 = Divide(x=w194, y=2.0) -> (x/y=w192:dbl)
              "Stroke Length _m_" <- w192
              n72 = Multiply(x=w186, y=w188) -> (x*y=w184:dbl)
              n73 = Multiply(x=w191, y=w192) -> (x*y=w190:dbl)
              "Charicteristic Velocity m_s" <- w190
              n74 = Multiply(x=w190, y=w187) -> (x*y=w189:dbl)
              n75 = Divide(x=w189, y=w185) -> (x/y=w182:dbl)
              "Reynolds Number" <- w182
              n76 = Divide(x=w184, y=w185) -> (x/y=w183:dbl)
              n77 = Square Root(x=w183) -> (sqrt(x)=w180:dbl)
              "Stokes Number" <- w180
              n78 = Square(x=w180) -> (x^2=w181:dbl)
              n79 = Divide(x=w181, y=w182) -> (x/y=→"Strouhal Number":dbl)
              "Velocity m_s" <- w198
              "RMS Velocity m_s" <- w203
              "Max Velocity m_s" <- w202
            }
            frame "RV (Vdi)" {
              n80 = Subtract(x=w204, y=w205) -> (x-y=→"Phase Displ _deg_":dbl)
              "Displacement _m_" <- w209
              "Max Displacement _m_" <- w207
              "RMS Dispacement _m_" <- w208
            }
            frame "Mano (Pressure)" {
              n81 = Subtract(x=w212, y=w211) -> (x-y=→"Phase Pressure _deg_":dbl)
              "Pressure _Pa_" <- w215
              "RMS Pressure _Pa_" <- w214
              "Max Pressure _Pa_" <- w213
            }
            frame "RV (Pressure)" {
              n82 = Subtract(x=w218, y=w217) -> (x-y=→"RV Phase Pressure _deg_":dbl)
              "RV Pressure _V_" <- w221
              "RV Max Pressure _V_" <- w219
              "RV RMS Pressure _V_" <- w220
            }
            frame "Pitot (Pitot)" {
            }
            frame "Gen (Current)" {
              n83 = Multiply(x=w232, y=w231) -> (x*y=w230:dbl[])
              n84 = Multiply(x=w238, y=w239) -> (x*y=w234:dbl[])
              "Power_W_" <- w234
              n85 = call "SJ_Get_Signal_Phase.vi"("No of Analogue Samples"=w227, "Number of Cycles"=w228, "Actual Sampling Frequency"=w229, "Signal"=w230) -> ("Phase Angle _deg_"=w226:dbl)  [unwired: 7 in]
              n86 = Subtract(x=w222, y=w224) -> (x-y=→"Phase Current _deg_":dbl)
              n87 = Subtract(x=w222, y=w226) -> (x-y=→"Phase Power _deg_":dbl)
              n88 = call-poly <vilib>:"RMS.vi"("X"=w234) -> ("rms value"=→"RMS Power _W_":dbl)  [unwired: 1 out]
              n89 = Array Max & Min(array=w234) -> (max value=→"Max Power _W_":dbl)  [unwired: 3 out]
              "Current _A_" <- w238
              "RMS Current _A_" <- w236
              "Max Current _A_" <- w235
            }
            frame "No Match", Default {
              n90 = One Button Dialog(message="Error in Signal Analysis", button name ("OK")="STOP") -> (true=w241:bool)
              n91 = Stop(stop? (T)=w241) -> ()
            }
          }
        }
        n92 = Divide(x=w123, y=w114) -> (x/y=w116:dbl)
        n93 = Divide(x=w118, y=w114) -> (x/y=w115:dbl)
        n94 = Subtract(x=w126, y=0.006) -> (x-y=w124:dbl)
        n95 = Subtract(x=w116, y=w124) -> (x-y=w122:dbl)
        n96 = Divide(x=w113, y=2.0) -> (x/y=w119:dbl)
        n97 = Divide(x=w122, y=w113) -> (x/y=→"DL:Streamwise:Position":dbl)
        n98 = Divide(x=w115, y=w119) -> (x/y=→"DL:Radius":dbl)
      }
      frame "LEM Calculations" {
        n99 = local read "Strouhal Number"() -> (w246:dbl)
        n100 = Reciprocal(x=w246) -> (1/x=w245:dbl)
        "Formation Criteria" <- w245
        n101 = Greater?(x=w245, y=0.16) -> (0:→"Jet Formation":bool)
        n102 = call "Read_Chan_Value_Gen.vi"("Desired Ch Names"=string[] ["Froude:NPL:Atmos_Press", "Aero_Tunnel:SmAD:Temp"], "Raw data file"=w249) -> ("Values"=w247:string[])  [unwired: 9 in]
        n103 = local read "Phase Pressure _deg_"() -> (w259:dbl)
        n104 = local read "Max Pressure _Pa_"() -> (w260:dbl)
        n105 = Fract/Exp String To Number(string=w247) -> (number=w268:dbl[])  [unwired: 3 in, 1 out]
        n106 = local read "Frequency (Hz)"() -> (w258:dbl)
        n107 = local read "Samps per cyle"() -> (w257:i32)
        n108 = Index Array(array=w268) -> (element #1=w265:dbl, element #2=w267:dbl)  [unwired: 2 in]
        n109 = Multiply(x=100.0 ("y"), y=w265) -> (x*y=w263:dbl)
        n110 = Add(x=w267, y=273.0) -> (x+y=w266:dbl)
        n111 = Bundle By Name(cluster=T8 {"R"=8.31451, "Mair"=0.0289645, "T"=293.0, "Patmos"=101325.0, "gamma"=1.4} ("Fluid Properties"), "Patmos"=w263, "T"=w266) -> (w261:T8)
        n112 = call "Get_LEM_Response.vi"("Frequency (Hz)"=w258, "Cavity Pressure Magnitude"=w260, "Cavity Pressure Phase"=w259, "Fluid Properties"=w261, "SJ Data IN"=w253) -> ("Phi"=w256:dbl, "Uo"=w255:dbl, "OmegaH"=w252:dbl)  [unwired: 2 in, 2 out]
        "LEM Phase Velocity _deg_" <- w256
        "LEM Max Velocity _ms_" <- w255
        n113 = call <vilib>:"Sine Pattern.vi"("phase(degrees)"=w256, "amplitude"=w255, "samples"=w257) -> ("Sinusoidal Pattern"=→"LEM Velocity _ms_":dbl[])  [unwired: 1 in, 1 out]
        n114 = Divide(x=w252, y=6.283185307179586) -> (x/y=→"Cavity:Helmholtz:Hz":dbl)
      }
      frame "Collect Mean Data" {
        n115 = local read "Samps per cyle"() -> (w339:i32)
        n116 = local read "Phase Average?"() -> (w274:bool)
        n117 = case shown="True" w274 {
          tunnel: [w379 w392] -> w349
          tunnel: [w378 w391] -> w348
          tunnel: [w377 w390] -> w347
          tunnel: [w376 w389] -> w346
          tunnel: [w375 w388] -> w345
          tunnel: [w374 w387] -> w344
          tunnel: [w373 w386] -> w343
          tunnel: [w372 w385] -> w340
          tunnel: [w371 w384] -> w336
          tunnel: [w370 w383] -> w317
          tunnel: [w369 w382] -> w316
          tunnel: [w368 w381] -> w280
          tunnel: [w367 w380] -> w277
          frame True {
            n118 = local read "LEM Phase Velocity _deg_"() -> (w369:dbl)
            n119 = local read "LEM Max Velocity _ms_"() -> (w370:dbl)
            n120 = local read "Max Displacement _m_"() -> (w375:dbl)
            n121 = local read "Formation Criteria"() -> (w372:dbl)
            n122 = local read "Phase Pressure _deg_"() -> (w377:dbl)
            n123 = local read "Max Power _W_"() -> (w376:dbl)
            n124 = local read "Phase Velocity _deg_"() -> (w378:dbl)
            n125 = local read "Phase Current _deg_"() -> (w379:dbl)
            n126 = local read "Max Pressure _Pa_"() -> (w371:dbl)
            n127 = local read "Max Velocity m_s"() -> (w373:dbl)
            n128 = local read "Max Current _A_"() -> (w374:dbl)
            n129 = local read "Reynolds Number"() -> (w367:dbl)
            n130 = local read "Jet Formation"() -> (w368:bool)
          }
          frame False {
            n131 = local read "LEM Max Velocity _ms_"() -> (w383:dbl)
            n132 = local read "Max Displacement _m_"() -> (w388:dbl)
            n133 = local read "RMS Dispacement _m_"() -> (w390:dbl)
            n134 = local read "RMS Velocity m_s"() -> (w385:dbl)
            n135 = local read "Max Power _W_"() -> (w389:dbl)
            n136 = local read "Strouhal Number"() -> (w382:dbl)
            n137 = local read "RMS Pressure _Pa_"() -> (w392:dbl)
            n138 = local read "Max Pressure _Pa_"() -> (w384:dbl)
            n139 = local read "RMS Power _W_"() -> (w391:dbl)
            n140 = local read "Max Velocity m_s"() -> (w386:dbl)
            n141 = local read "Max Current _A_"() -> (w387:dbl)
            n142 = local read "Reynolds Number"() -> (w380:dbl)
            n143 = local read "Jet Formation"() -> (w381:bool)
          }
        }
        n144 = call-poly <vilib>:"Ramp Pattern.vi"("exclude end?"=TRUE, "start"=0.0, "end"=360.0, "samples"=w339) -> ("Ramp Pattern"=w292:dbl[])  [unwired: 6 in, 1 out]
        "Phase Angle _deg_" <- w292
        n145 = local read "LEM Velocity _ms_"() -> (w288:dbl[])
        n146 = local read "Input Voltage _V_"() -> (w326:dbl[])
        n147 = local read "Displacement _m_"() -> (w319:dbl[])
        n148 = local read "Velocity m_s"() -> (w285:dbl[])
        n149 = local read "Pressure _Pa_"() -> (w324:dbl[])
        n150 = call "Get_Variable_Name.vi"("Data"=w317) -> ("Data Name(s)"=w314:string[], "Data Values(s)"=w295:string[])  [unwired: 24 in, 1 out]
        n151 = call "Get_Variable_Name.vi"("Data"=w336) -> ("Data Name(s)"=w305:string[], "Data Values(s)"=w304:string[])  [unwired: 24 in, 1 out]
        n152 = call "Get_Variable_Name.vi"("Data"=w343) -> ("Data Name(s)"=w306:string[], "Data Values(s)"=w303:string[])  [unwired: 24 in, 1 out]
        n153 = call "Get_Variable_Name.vi"("Data"=w344) -> ("Data Name(s)"=w307:string[], "Data Values(s)"=w302:string[])  [unwired: 24 in, 1 out]
        n154 = call "Get_Variable_Name.vi"("Data"=w345) -> ("Data Name(s)"=w308:string[], "Data Values(s)"=w301:string[])  [unwired: 24 in, 1 out]
        n155 = call "Get_Variable_Name.vi"("Data"=w346) -> ("Data Name(s)"=w309:string[], "Data Values(s)"=w300:string[])  [unwired: 24 in, 1 out]
        n156 = call "Get_Variable_Name.vi"("Data"=w347) -> ("Data Name(s)"=w310:string[], "Data Values(s)"=w299:string[])  [unwired: 24 in, 1 out]
        n157 = call "Get_Variable_Name.vi"("Data"=w348) -> ("Data Name(s)"=w311:string[], "Data Values(s)"=w298:string[])  [unwired: 24 in, 1 out]
        n158 = call "Get_Variable_Name.vi"("Data"=w349) -> ("Data Name(s)"=w312:string[], "Data Values(s)"=w297:string[])  [unwired: 24 in, 1 out]
        n159 = call "Get_Variable_Name.vi"("Data"=w340) -> ("Data Name(s)"=w313:string[], "Data Values(s)"=w296:string[])  [unwired: 24 in, 1 out]
        n160 = call "Get_Variable_Name.vi"("Data"=w316) -> ("Data Name(s)"=w315:string[], "Data Values(s)"=w294:string[])  [unwired: 24 in, 1 out]
        n161 = call "Get_Variable_Name.vi"("Data"=w280) -> ("Data Name(s)"=w279:string[], "Data Values(s)"=w278:string[])  [unwired: 24 in, 1 out]
        n162 = call "Get_Variable_Name.vi"("Data"=w277) -> ("Data Name(s)"=w276:string[], "Data Values(s)"=w275:string[])  [unwired: 24 in, 1 out]
        n163 = local read "Current _A_"() -> (w321:dbl[])
        n164 = Build Array(w304, w303, w302, w301, w300, w299, w298, w297, w296, w295, w294, w279, w276) -> (w335:string[][])
        n165 = call-poly <vilib>:"Quick Scale.vi"("X"=w288) -> ("Y[i]=X[i]/Max|X|"=w286:dbl[], "max|X|"=w287:dbl)  [unwired: 1 out]
        n166 = local read "Cavity:Helmholtz:Hz"() -> (w282:dbl)
        n167 = call-poly <vilib>:"Quick Scale.vi"("X"=w326) -> ("Y[i]=X[i]/Max|X|"=w325:dbl[])  [unwired: 2 out]
        n168 = call-poly <vilib>:"Quick Scale.vi"("X"=w324) -> ("Y[i]=X[i]/Max|X|"=w323:dbl[])  [unwired: 2 out]
        n169 = call-poly <vilib>:"Quick Scale.vi"("X"=w319) -> ("Y[i]=X[i]/Max|X|"=w322:dbl[])  [unwired: 2 out]
        n170 = call-poly <vilib>:"Quick Scale.vi"("X"=w321) -> ("Y[i]=X[i]/Max|X|"=w320:dbl[])  [unwired: 2 out]
        n171 = Build Array(w305, w306, w307, w308, w309, w310, w311, w312, w313, w314, w315, w278, w275) -> (w293:string[][])
        n172 = local read "Frequency (Hz)"() -> (w283:dbl)
        n173 = Divide(x=w285, y=w287) -> (x/y=w284:dbl[])
        n174 = local read "Amplitude (V)"() -> (w351:dbl)
        n175 = for {
          tunnel: w335 -> [w397] mode=indexing
          tunnel: [w395] -> w332 mode=indexing
          n176 = Index Array(array=w397) -> (element=w396:string)  [unwired: 1 in]
          n177 = Fract/Exp String To Number(string=w396) -> (number=w395:dbl)  [unwired: 3 in, 1 out]
        }
        n178 = Bundle("Ramp Pattern"=w292, "Y[i]=X[i]/Max|X|"=w325) -> (w354:T11)  [unwired: 1 in]
        n179 = Bundle("Ramp Pattern"=w292, "Y[i]=X[i]/Max|X|"=w323) -> (w363:T11)  [unwired: 1 in]
        n180 = Bundle("Ramp Pattern"=w292, "Y[i]=X[i]/Max|X|"=w322) -> (w364:T11)  [unwired: 1 in]
        n181 = Bundle("Ramp Pattern"=w292, "Y[i]=X[i]/Max|X|"=w320) -> (w353:T11)  [unwired: 1 in]
        n182 = Bundle("Ramp Pattern"=w292, w284) -> (w365:cluster{"Ramp Pattern":dbl[], dbl[]})  [unwired: 1 in]
        n183 = Bundle("Ramp Pattern"=w292, "Y[i]=X[i]/Max|X|"=w286) -> (w318:T11)  [unwired: 1 in]
        n184 = for {
          tunnel: w293 -> [w394] mode=indexing
          tunnel: [w393] -> w290 mode=indexing
          n185 = Index Array(array=w394) -> (element=w393:string)  [unwired: 1 in]
        }
        "Output Data Names" <- w290
        n186 = Divide(x=w283, y=w282) -> (x/y=w281:dbl)
        "DL:Frequency" <- w281
        n187 = Build Array(w354, w363) -> (→"Pressure Plot":T12)
        n188 = Build Array(w354, w364) -> (→"Displacement Plot":T12)
        n189 = Build Array(w354, w353) -> (→"Current Plot":T12)
        n190 = Build Array(w354, w365, w318) -> (→"Velocity Plot":T12)
        n191 = Build Array(w281, w351) -> (w331:dbl[])
        n192 = property on="Menu Ring" class="Ring (strict)"("Strings []"=w290) -> ()  [unwired: 2 in, 2 out]
        n193 = Index Array(array=w290, index=w333) -> (element=w342:string)
        n194 = Insert Into Array(array=w332, index=0, new element=w331) -> (w330:dbl[])
        n195 = property on="Pressure v Frequency" class="XYGraph (strict)"("YScale.NameLbl.Text"=w342) -> ()  [unwired: 2 in, 2 out]
        n196 = Add(x=u16 2, y=w333) -> (x+y=w341:u16)
        n197 = Build Array (concatenate)(w359, w330) -> (w358:dbl[][])
        n198 = Index Array(array=w358, index (col) #1=0 ("disabled index (col)"), index (col) #2=w341) -> (element #1=w356:dbl[], element #2=w350:dbl[])  [unwired: 2 in]
        n199 = Bundle(w356, w350) -> (→"Pressure v Frequency":cluster{dbl[], dbl[]})  [unwired: 1 in]
      }
      frame "Save Phase Average File" {
        w466 = 0 ("No of Bins")
        n200 = local read "Phase Angle _deg_"() -> (w457:dbl[])
        n201 = local read "LEM Velocity _ms_"() -> (w425:dbl[])
        n202 = local read "Input Voltage _V_"() -> (w490:dbl[])
        n203 = local read "Displacement _m_"() -> (w489:dbl[])
        n204 = local read "DL:Streamwise:Position"() -> (w411:dbl)
        n205 = local read "LEM Max Velocity _ms_"() -> (w421:dbl)
        n206 = Strip Path(path=w474) -> (stripped path=w478:path)  [unwired: 1 out]
        n207 = local read "Pressure _Pa_"() -> (w486:dbl[])
        n208 = local read "Cavity:Helmholtz:Hz"() -> (w404:dbl)
        n209 = local read "Max Pressure _Pa_"() -> (w469:dbl)
        n210 = local read "Current _A_"() -> (w488:dbl[])
        n211 = local read "Velocity m_s"() -> (w485:dbl[])
        n212 = local read "Max Velocity m_s"() -> (w422:dbl)
        n213 = local read "Power_W_"() -> (w487:dbl[])
        n214 = local read "Frequency (Hz)"() -> (w403:dbl)
        n215 = local read "DL:Frequency"() -> (w471:dbl)
        n216 = local read "Amplitude (V)"() -> (w470:dbl)
        n217 = Strip Path(path=w478) -> (stripped path=w480:path, name=w483:string)
        n218 = local read "DL:Radius"() -> (w412:dbl)
        n219 = Strip Path(path=w480) -> (stripped path=w479:path)  [unwired: 1 out]
        n220 = Concatenate Strings(w483, "_" ("string"), w415, ".xls" ("string")) -> (w484:string)
        n221 = Strip Path(path=w479) -> (stripped path=w481:path)  [unwired: 1 out]
        n222 = call "Get_Variable_Name.vi"("Data"=w457) -> ("Data Name(s)"=w441:string[], "Data Values(s)"=w428:string[])  [unwired: 24 in, 1 out]
        n223 = call "Get_Variable_Name.vi"("Data"=w425) -> ("Data Name(s)"=w424:string[], "Data Values(s)"=w423:string[])  [unwired: 24 in, 1 out]
        n224 = call "Get_Variable_Name.vi"("Data"=w490) -> ("Data Name(s)"=w446:string[], "Data Values(s)"=w436:string[])  [unwired: 24 in, 1 out]
        n225 = call "Get_Variable_Name.vi"("Data"=w489) -> ("Data Name(s)"=w445:string[], "Data Values(s)"=w435:string[])  [unwired: 24 in, 1 out]
        n226 = call "Get_Variable_Name.vi"("Data"=w488) -> ("Data Name(s)"=w444:string[], "Data Values(s)"=w434:string[])  [unwired: 24 in, 1 out]
        n227 = call "Get_Variable_Name.vi"("Data"=w487) -> ("Data Name(s)"=w443:string[], "Data Values(s)"=w433:string[])  [unwired: 24 in, 1 out]
        n228 = call "Get_Variable_Name.vi"("Data"=w486) -> ("Data Name(s)"=w431:string[], "Data Values(s)"=w430:string[])  [unwired: 24 in, 1 out]
        n229 = call "Get_Variable_Name.vi"("Data"=w485) -> ("Data Name(s)"=w442:string[], "Data Values(s)"=w432:string[])  [unwired: 24 in, 1 out]
        n230 = call "Get_Variable_Name.vi"("Data"=w415) -> ("Data Name(s)"=w456:string[], "Data Values(s)"=w450:string[])  [unwired: 24 in, 1 out]
        n231 = call "Get_Variable_Name.vi"("Data"=w471) -> ("Data Name(s)"=w455:string[], "Data Values(s)"=w449:string[])  [unwired: 24 in, 1 out]
        n232 = call "Get_Variable_Name.vi"("Data"=w470) -> ("Data Name(s)"=w454:string[], "Data Values(s)"=w448:string[])  [unwired: 24 in, 1 out]
        n233 = call "Get_Variable_Name.vi"("Data"=w469) -> ("Data Name(s)"=w453:string[], "Data Values(s)"=w447:string[])  [unwired: 24 in, 1 out]
        n234 = call "Get_Variable_Name.vi"("Data"=w422) -> ("Data Name(s)"=w420:string[], "Data Values(s)"=w418:string[])  [unwired: 24 in, 1 out]
        n235 = call "Get_Variable_Name.vi"("Data"=w421) -> ("Data Name(s)"=w419:string[], "Data Values(s)"=w417:string[])  [unwired: 24 in, 1 out]
        n236 = call "Get_Variable_Name.vi"("Data"=w411) -> ("Data Name(s)"=w408:string[], "Data Values(s)"=w410:string[])  [unwired: 24 in, 1 out]
        n237 = call "Get_Variable_Name.vi"("Data"=w412) -> ("Data Name(s)"=w407:string[], "Data Values(s)"=w409:string[])  [unwired: 24 in, 1 out]
        n238 = call "Get_Variable_Name.vi"("Data"=w404) -> ("Data Name(s)"=w406:string[], "Data Values(s)"=w405:string[])  [unwired: 24 in, 1 out]
        n239 = call "Get_Variable_Name.vi"("Data"=w403) -> ("Data Name(s)"=w402:string[], "Data Values(s)"=w401:string[])  [unwired: 24 in, 1 out]
        n240 = Build Path(base path=w481, name or relative path="Results_Post_Processed") -> (appended path=w477:path)
        n241 = Build Path(base path=w477, name or relative path="Phase_Averaged" ("New Results Folder Name")) -> (appended path=w476:path)
        n242 = Build Array(w446, w445, w444, w443, w431, w442, w424) -> (w438:string[][])
        n243 = Build Path(base path=w476, name or relative path=w484) -> (appended path=w460:path)
        n244 = local read "Samps per cyle"() -> (w458:i32)
        n245 = for {
          tunnel: w438 -> [w492] mode=indexing
          tunnel: [w491] -> w437 mode=indexing
          n246 = Index Array(array=w492) -> (element=w491:string)  [unwired: 1 in]
        }
        n247 = Build Array(w436, w435, w434, w433, w430, w432, w423) -> (w429:string[][])
        n248 = call <vilib>:"Check if File or Folder Exists.vi"("path"=w460) -> ("file or folder exists?"=w398:bool, "dup path"=w399:path)  [unwired: 8 in, 1 out]
        n249 = Build Array(w456, w455, w454, w453, w420, w419, w408, w407, w406, w402) -> (w452:string[][])
        n250 = Array Size(array=w437) -> (size(s)=w459:i32)
        n251 = Build Array(w450, w449, w448, w447, w418, w417, w410, w409, w405, w401) -> (w468:string[][])
        n252 = Index Array(array=w441) -> (element=w440:string)  [unwired: 1 in]
        n253 = Compound Arithmetic op=MULTIPLY(w458, w459) -> (w439:i32)
        n254 = for {
          tunnel: w452 -> [w494] mode=indexing
          tunnel: [w493] -> w451 mode=indexing
          n255 = Index Array(array=w494) -> (element=w493:string)  [unwired: 1 in]
        }
        n256 = for {
          tunnel: w468 -> [w496] mode=indexing
          tunnel: [w495] -> w465 mode=indexing
          n257 = Index Array(array=w496) -> (element=w495:string)  [unwired: 1 in]
        }
        n258 = for {
          N: w439 -> [_]
          tunnel: w437 -> [w508]
          shift-right: [w511] -> _
          shift-left: w466 -> [w504]
          tunnel: w458 -> [w512]
          tunnel: w428 -> [w506]
          tunnel: [w497] -> w467 mode=indexing
          tunnel: w429 -> [w507]
          shift-right: [w505] -> _
          shift-left: w466 -> [w503]
          tunnel: [w502] -> w464 mode=indexing
          tunnel: w440 -> [w500]
          w499 = ":"
          n259 = Index Array(array=w508, index=w503) -> (element=w501:string)
          n260 = Index Array(array=w507, index (row)=w503, index (col)=w504) -> (element=w502:string)
          n261 = Index Array(array=w506, index=w504) -> (element=w498:string)
          n262 = Increment(x=w504) -> (x+1=w510:i32)
          n263 = Concatenate Strings(w501, w499, w500, w499, w498) -> (w497:string)
          n264 = Equal?(x=w512, y=w510) -> (x = y?=w509:bool)
          n265 = case shown="True" w509 {
            tunnel: [w514 0] -> w511
            tunnel: w510 -> [w514 _]
            tunnel: w503 -> [w513 w516]
            tunnel: [w513 w515] -> w505
            frame False {
            }
            frame True {
              n266 = Increment(x=w516) -> (x+1=w515:i32)
            }
          }
        }
        n267 = Insert Into Array(array=w465, new element=w464) -> (w461:string[])  [unwired: 1 in]
        n268 = Insert Into Array(array=w451, new element=w467) -> (w463:string[])  [unwired: 1 in]
        n269 = Build Array(w461) -> (w462:string[][])
        n270 = call "Write_Ch_data_file.vi"("Append last row only"=FALSE, "exists?"=w398, "Channel Values"=w462, "Channel names"=w463, "Filename"=w399) -> ()  [unwired: 7 in]
      }
      frame "Save Mean Data" {
        n271 = local read "DL:Streamwise:Position"() -> (w548:dbl)
        n272 = local read "Output Data Names"() -> (w573:string[])
        n273 = local read "Cavity:Helmholtz:Hz"() -> (w528:dbl)
        n274 = Build Array("Aero_Tunnel:Abs Pressure:Bar" ("element")) -> (w523:string[])
        n275 = Array Subset(array=w570, index (col)=2 ("index")) -> (w574:dbl[][])  [unwired: 3 in]
        n276 = call "Read_Chan_Value_Gen.vi"("Desired Ch Names"=w523, "Raw data file"=w525) -> ("Values"=w522:string[])  [unwired: 9 in]
        n277 = Unbundle By Name(w569) -> ("Do"=w568:dbl, "Dc"=w567:dbl, "Ho"=w566:dbl, "Hc"=w565:dbl, "K"=w564:dbl, "beta"=w563:dbl)
        n278 = local read "DL:Radius"() -> (w547:dbl)
        n279 = Index Array(array=w522) -> (element=w521:string)  [unwired: 1 in]
        n280 = Index Array(array=w570, index (col) #1=1 ("disabled index (col)"), index (col) #2=0 ("index (col)")) -> (element #1=w552:dbl[], element #2=w551:dbl[])  [unwired: 2 in]
        n281 = Build Array(w521) -> (w541:string[])
        n282 = Build Array("Atmospheric Pressure:Pa" ("string")) -> (w542:string[])
        n283 = Build Array(w544) -> (w540:string[])
        n284 = Build Array("Comment:String" ("string")) -> (w562:string[])
        n285 = call "Get_Variable_Name.vi"("Data"=w568) -> ("Data Name(s)"=w561:string[], "Data Values(s)"=w539:string[])  [unwired: 24 in, 1 out]
        n286 = call "Get_Variable_Name.vi"("Data"=w567) -> ("Data Name(s)"=w560:string[], "Data Values(s)"=w538:string[])  [unwired: 24 in, 1 out]
        n287 = call "Get_Variable_Name.vi"("Data"=w566) -> ("Data Name(s)"=w559:string[], "Data Values(s)"=w537:string[])  [unwired: 24 in, 1 out]
        n288 = call "Get_Variable_Name.vi"("Data"=w565) -> ("Data Name(s)"=w558:string[], "Data Values(s)"=w536:string[])  [unwired: 24 in, 1 out]
        n289 = call "Get_Variable_Name.vi"("Data"=w564) -> ("Data Name(s)"=w557:string[], "Data Values(s)"=w535:string[])  [unwired: 24 in, 1 out]
        n290 = call "Get_Variable_Name.vi"("Data"=w563) -> ("Data Name(s)"=w556:string[], "Data Values(s)"=w534:string[])  [unwired: 24 in, 1 out]
        n291 = call "Get_Variable_Name.vi"("Data"=w548) -> ("Data Name(s)"=w546:string[], "Data Values(s)"=w533:string[])  [unwired: 24 in, 1 out]
        n292 = call "Get_Variable_Name.vi"("Data"=w547) -> ("Data Name(s)"=w545:string[], "Data Values(s)"=w532:string[])  [unwired: 24 in, 1 out]
        n293 = call "Get_Variable_Name.vi"("Data"=w528) -> ("Data Name(s)"=w527:string[], "Data Values(s)"=w526:string[])  [unwired: 24 in, 1 out]
        n294 = for {
          tunnel: w525 -> [w611]
          tunnel: w573 -> [w610] mode=indexing
          tunnel: [w608] -> w572 mode=indexing
          tunnel: [w607] -> w571 mode=indexing
          n295 = call "Get_New_Path_from_raw_data.vi"("New Results File Name"=w610, "New Results Folder Name"="_Mean_Data" ("string"), "Raw data file"=w611) -> ("Does it already exist?"=w608:bool, "New Spreadsheet Results File"=w607:path)  [unwired: 7 in]
        }
        n296 = for {
          tunnel: "Amp & Freq:" ("string") -> [w590]
          tunnel: w552 -> [w589] mode=indexing
          tunnel: w551 -> [w585] mode=indexing
          tunnel: [w583] -> w549 mode=indexing
          w584 = i16 3 ("precision (6)")
          n297 = Number To Fractional String(number=w589, precision (6)=w584) -> (F-format string=w588:string)  [unwired: 2 in]
          n298 = Number To Fractional String(number=w585, precision (6)=w584) -> (F-format string=w586:string)  [unwired: 2 in]
          n299 = Concatenate Strings(w590, w588, ":" ("string"), w586) -> (w583:string)
        }
        n300 = Build Array(w542, w562, w561, w560, w559, w558, w557, w556, w546, w545, w527) -> (w555:string[][])
        n301 = Build Array(w541, w540, w539, w538, w537, w536, w535, w534, w533, w532, w526) -> (w531:string[][])
        n302 = for {
          tunnel: w555 -> [w592] mode=indexing
          tunnel: [w591] -> w550 mode=indexing
          n303 = Index Array(array=w592) -> (element=w591:string)  [unwired: 1 in]
        }
        n304 = for {
          tunnel: w531 -> [w582] mode=indexing
          tunnel: [w581] -> w530 mode=indexing
          n305 = Index Array(array=w582) -> (element=w581:string)  [unwired: 1 in]
        }
        n306 = Insert Into Array(array=w550, new element=w549) -> (w529:string[])  [unwired: 1 in]
        n307 = for {
          tunnel: w574 -> [w603]
          tunnel: w572 -> [w601] mode=indexing
          tunnel: w571 -> [w599] mode=indexing
          tunnel: w530 -> [w597]
          tunnel: w529 -> [w593]
          i -> [w602]
          n308 = Index Array(array=w603, index (col)=w602) -> (element=w598:dbl[])  [unwired: 1 in]
          n309 = for {
            tunnel: w598 -> [w606] mode=indexing
            tunnel: [w605] -> w596 mode=indexing
            n310 = Number To Fractional String(number=w606, precision (6)=i16 7) -> (F-format string=w605:string)  [unwired: 2 in]
          }
          n311 = Insert Into Array(array=w597, new element=w596) -> (w595:string[])  [unwired: 1 in]
          n312 = Build Array(w595) -> (w594:string[][])
          n313 = call "Write_Ch_data_file.vi"("Append last row only"=FALSE, "exists?"=w601, "Channel Values"=w594, "Channel names"=w593, "Filename"=w599) -> ()  [unwired: 7 in]
        }
        n314 = call "Ch_Active_Control_Client.vi"("Match"="Synthetic_Jet", "Activate Channels?"=FALSE, "Control on"=enum16{"Channel Name", "Main Address"}."Channel Name") -> ()  [unwired: 2 out]
      }
    }
  }
